vi "SLSC Get Capabilities from Custom Device.vi"(6 "Property Name":string="Capabilities", 8 "error in (no error)":errorcluster, 10 "Default Value":T1={"vendorNum"=0, "vendorName"="", "vendorPrefix"="", "productNum"=0, "productName"="", "capsVersion"="", "capsSpecVersion"=0, "capsSpecOldestCompatibleVersion"=1, "enums"=[], "properties"=[], "commands"=[], "scales"=[], "physicalChannels"=[], "registerMap"={"registers"=[]}}, 11 "Device Item Ref in":T8 format="%.0x") -> (0 "error out":errorcluster, 1 "Product Name":string, 2 "data":T1={"vendorNum"=0, "vendorName"="", "vendorPrefix"="", "productNum"=0, "productName"="", "capsVersion"="", "capsSpecVersion"=0, "capsSpecOldestCompatibleVersion"=1, "enums"=[], "properties"=[], "commands"=[], "scales"=[], "physicalChannels"=[], "registerMap"={"registers"=[]}}, 3 "Item Ref out":T8=18446744073709551615 format="%.0x", 4 "Product Num":u32, 5 "Vendor Prefix":string)   [LabVIEW 2015, in "SLSC CD System Explorer.lvlib"]
uses:
  SLSC CD System Explorer.lvlib
  <vilib>/NI Veristand/Custom Device API/Custom Device Item Ref.ctl
  SLSC EDS API/JSON parsing/EDSjsonStructure.ctl
  SLSC EDS API/JSON parsing/enum.ctl
  SLSC EDS API/JSON parsing/property.ctl
  SLSC EDS API/JSON parsing/command.ctl
  SLSC EDS API/JSON parsing/scale.ctl
  SLSC EDS API/JSON parsing/physicalChannel.ctl
  SLSC EDS API/JSON parsing/register.ctl
  <vilib>/NI Veristand/Custom Device API/Get Item Property (Variant).vi
  <vilib>/NI VeriStand/Custom Device API/Custom Device API.lvlib
panel:
  out "Found?":bool
  # "not working\nregisterMap->registers->initialValue"
  # "not working\nregisterMap->registers->initialValue"
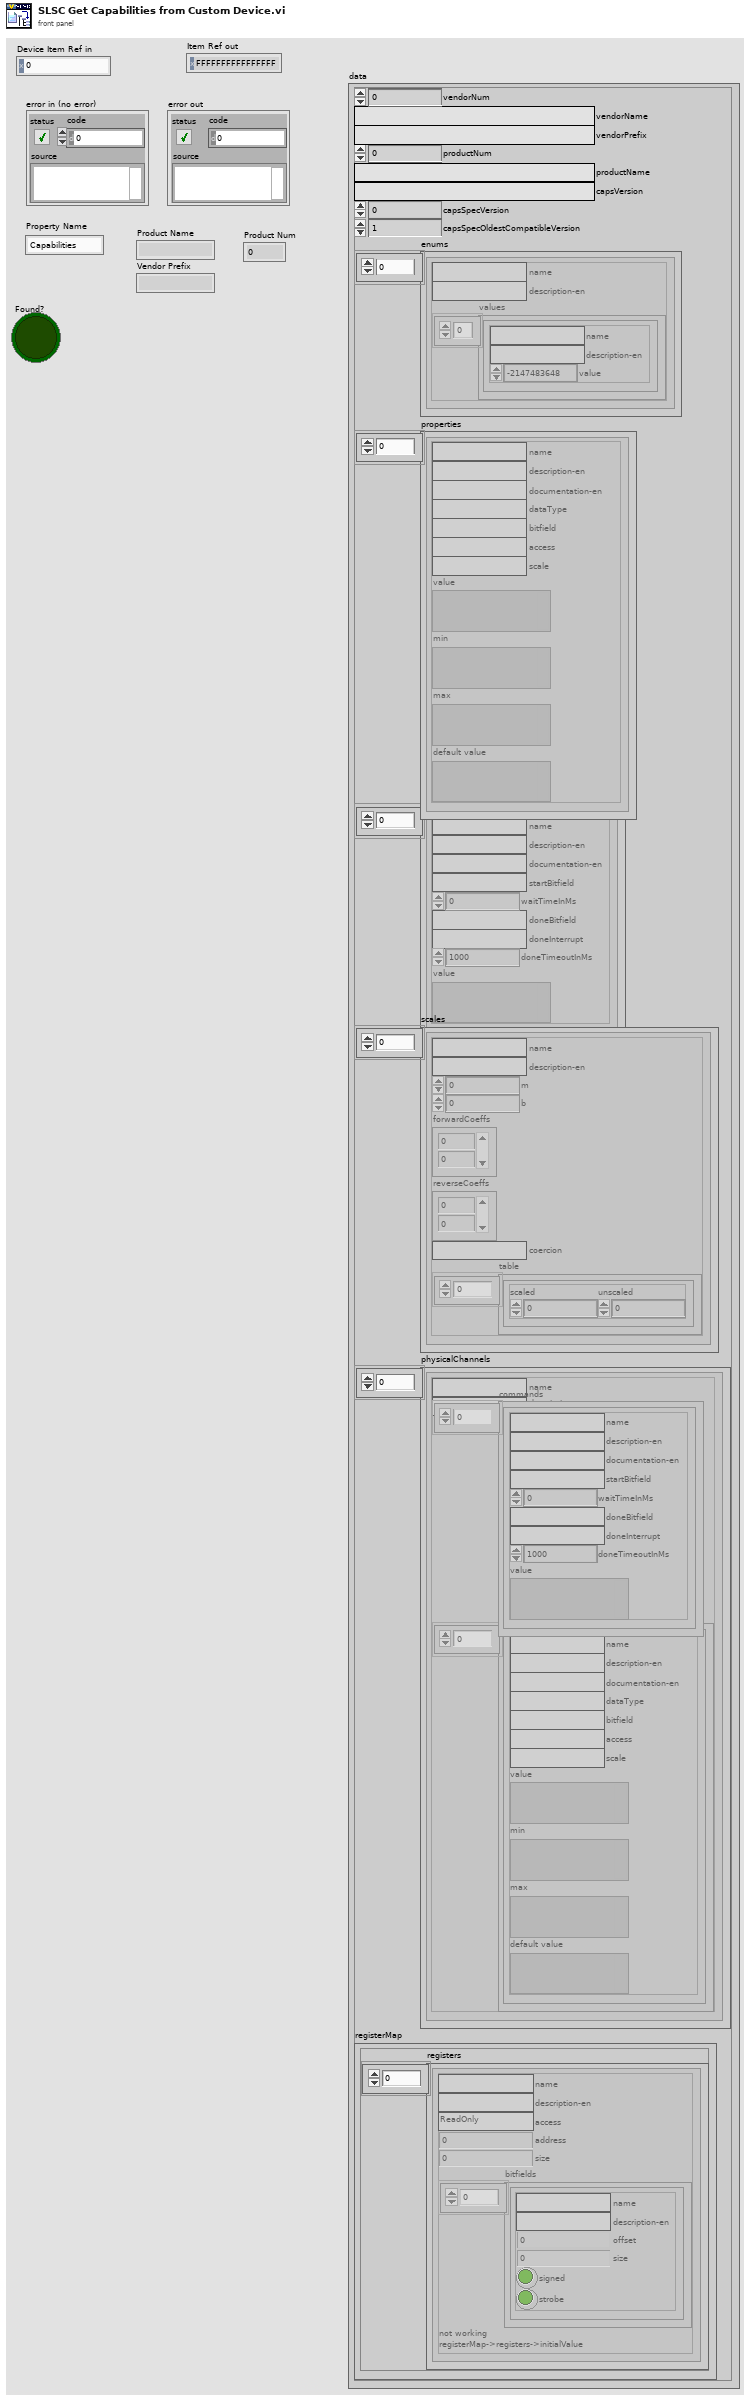
[diagram p1: front panel]
types:
  T1 = typedef "EDSjsonStructure.ctl" = cluster{"vendorNum":u32, "vendorName":string, "vendorPrefix":string, "productNum":u32, "productName":string, "capsVersion":string, "capsSpecVersion":u32, "capsSpecOldestCompatibleVersion":u32, "enums":T2[], "properties":T3[], "commands":T4[], "scales":T5[], "physicalChannels":T6[], "registerMap":cluster{"registers":T7[]}}
  T2 = typedef "enum.ctl" = cluster{"name":string, "description-en":string, "values":cluster{"name":string, "description-en":string, "value":i32}[]}
  T3 = typedef "property.ctl" = cluster{"name":string, "description-en":string, "documentation-en":string, "dataType":string, "bitfield":string, "access":string, "scale":string, "value":variant, "min":variant, "max":variant, "default value":variant}
  T4 = typedef "command.ctl" = cluster{"name":string, "description-en":string, "documentation-en":string, "startBitfield":string, "waitTimeInMs":i32, "doneBitfield":string, "doneInterrupt":string, "doneTimeoutInMs":i32, "value":variant}
  T5 = typedef "scale.ctl" = cluster{"name":string, "description-en":string, "m":dbl, "b":dbl, "forwardCoeffs":dbl[], "reverseCoeffs":dbl[], "coercion":string, "table":cluster{"scaled":dbl, "unscaled":dbl}[]}
  T6 = typedef "physicalChannel.ctl" = cluster{"name":string, "description-en":string, "commands":T4[], "properties":T3[]}
  T7 = typedef "register.ctl" = cluster{"name":string, "description-en":string, "access":string, "address":u32, "size":u32, "bitfields":cluster{"name":string, "description-en":string, "offset":u32, "size":u32, "signed":bool, "strobe":bool}[]}
  T8 = typedef "Custom Device API.lvlib/Custom Device Item Ref.ctl" = u64
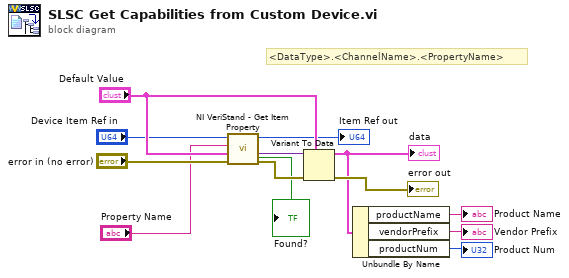
[diagram p0: block diagram]
diagram:
  # "<DataType>.<ChannelName>.<PropertyName>"
  n1 = call-poly <vilib>:"NI VeriStand - Get Item Property.vi"("error in (no error)"="error in (no error)", "Default Value"="Default Value", "Property Name"="Property Name", "Item Ref in"="Device Item Ref in") -> ("error out"=w8:errorcluster, "Value"=w13:variant, "Item Ref out"=→"Item Ref out":T8, "Found?"=→"Found?":bool)  [unwired: 4 in]
  n2 = Variant To Data(error in=w8, type="Default Value", Variant=w13) -> (data=w4:T1, error out=→"error out":errorcluster)
  "data" <- w4
  n3 = Unbundle By Name(w4) -> ("productName"=→"Product Name":string, "vendorPrefix"=→"Vendor Prefix":string, "productNum"=→"Product Num":u32)
